vi "getWaypoints.vi"(8 "error in (no error)":errorcluster, 11 "GoTo in":refnum<class "GoTo.lvclass">) -> (0 "error out":errorcluster, 2 "Waypoint Array":refnum<class "Waypoint.lvclass">[](array[class]), 3 "GoTo out":refnum<class "GoTo.lvclass">)   [LabVIEW 2013, in "GoTo.lvclass"]
uses:
  GoTo.lvclass
  Waypoint/Waypoint.lvclass
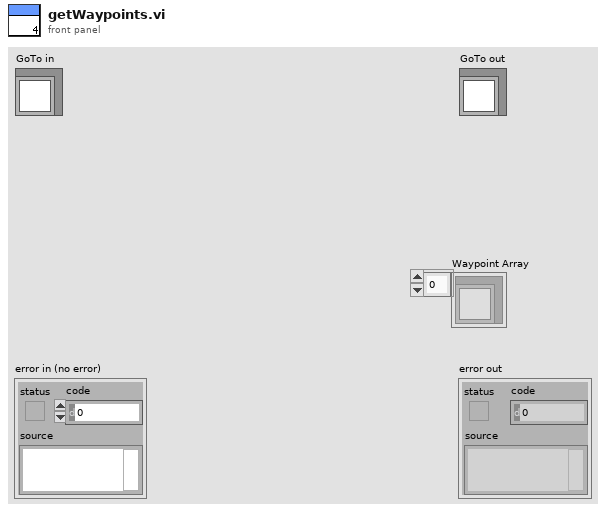
[diagram p1: front panel]
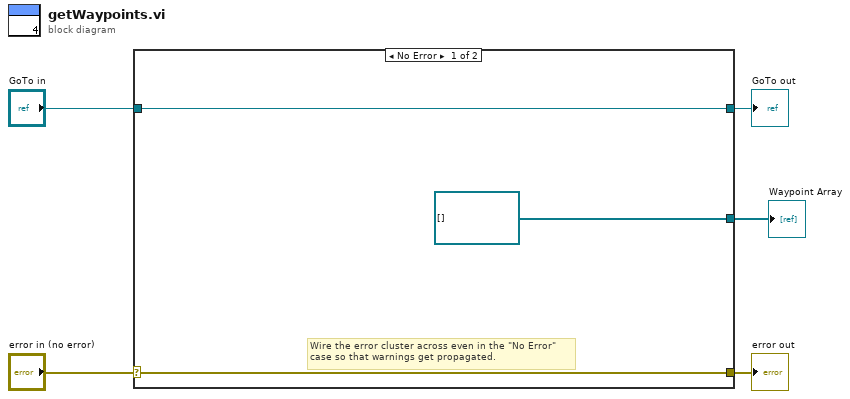
[diagram p0: block diagram]
diagram:
  n1 = case shown="No Error" "error in (no error)" {
    selector: "error in (no error)" -> [w7 w10]
    tunnel: [w7 w10] -> w4
    tunnel: [w8 w9] -> w2
    tunnel: "GoTo in" -> [w8 w9]
    tunnel: [refnum<class "Waypoint.lvclass">[] [] ("Array 2") _] -> w1
    frame No Error {
      # "Wire the error cluster across even in the \"No Error\"\ncase so that warnings get propagated."
    }
    frame Error {
    }
  }
  "error out" <- w4
  "GoTo out" <- w2
  "Waypoint Array" <- w1
